vi "RIB Req - UDP Normal Operation.vi"(0 "Limits File Path":path, 5 "Results File Path":path, 11 "error in":errorcluster) -> (4 "Results Data Array":string[][](array[string]), 15 "error out":errorcluster)   [LabVIEW 2024]
doc: "Template test"
uses:
  <vilib>/addons/_JKI Toolkits/State Machine/_JKI_lib_State_Machine.llb/Select State(s)_err__jki_lib_state_machine.vi
  <vilib>/addons/_JKI Toolkits/State Machine/_JKI_lib_State_Machine.llb/Select State(s)_bool__jki_lib_state_machine.vi
  <vilib>/addons/_JKI Toolkits/State Machine/_JKI_lib_State_Machine.llb/Periodic Trigger__ogtk__JKI-SM__jki_lib_state_machine.vi
  <userlib>/_OpenG.lib/file/file.llb/Strip Path Extension - String__ogtk.vi
  <vilib>/Utility/file.llb/Read Delimited Spreadsheet (string).vi
  <userlib>/_OpenG.lib/file/file.llb/openg_file.lvlib
  <userlib>/_OpenG.lib/appcontrol/appcontrol.llb/openg_application_control.lvlib
  <userlib>/_OpenG.lib/time/time.llb/openg_time.lvlib
  <vilib>/Utility/file.llb/Write Delimited Spreadsheet (string).vi
panel:
  in  "Connect":string
  in  "Connect Fail":string
  out "Normal Operation":bool
  out "Wait for Start":bool
  out "Timeout (Normal Operation)":dbl(slide) scale=0.0..10.0
  out "Timeout (Wait for Start)":dbl(slide) scale=0.0..10.0
  in  "Read Normal Operation":string
  in  "Read Wait for Start":string
  in  "Read TMS":string
  in  "Read ROV B":string
  in  "Read ROV A":string
  out "Results Data 10":string[](array[string])
  out "Results Data 9":string[](array[string])
  in  "5A Test":bool
  in  "task out":refnum<k21>
  in  "UDP Read":string
  in  "connection ID":refnum<k16>
  in  "Exit":bool
  # "Normal Operation Test"
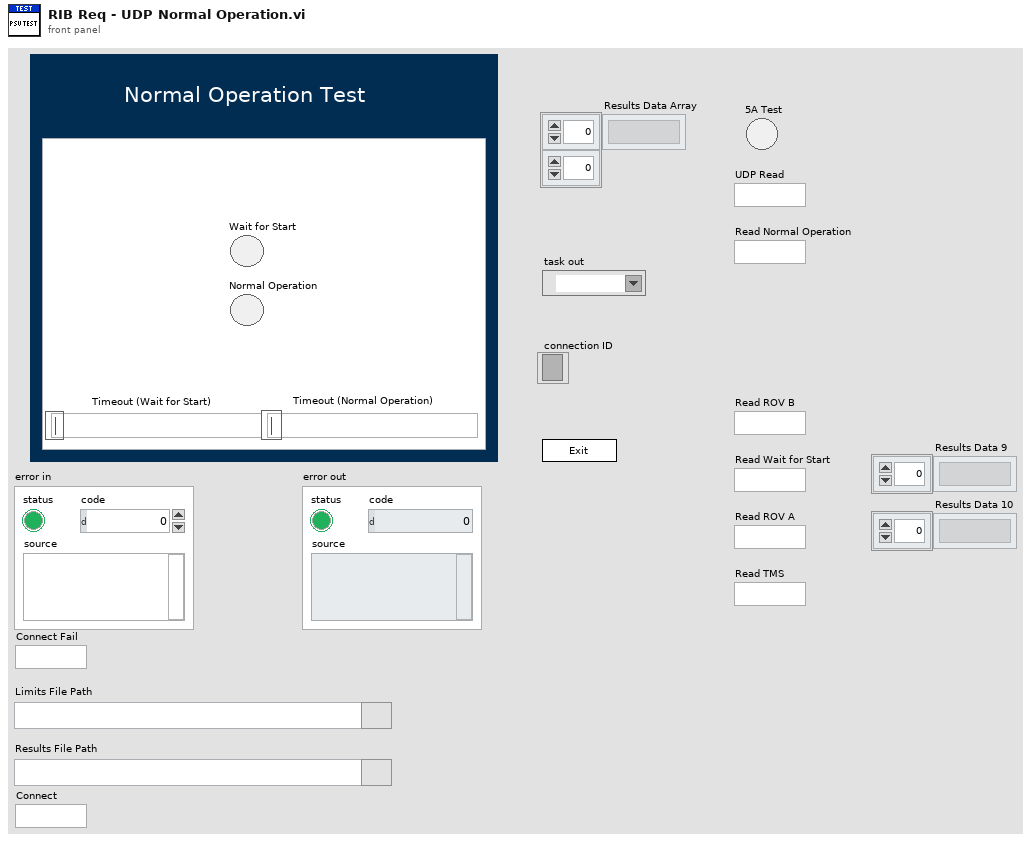
[diagram p1: front panel]
types:
  T1 = enum32{"Invalid", "Standard", "Closed", "Hidden", "Minimized", "Maximized"}
  T2 = enum32{"invalid app kind", "Development System", "Run Time System", "Student Edition", "Embedded LabVIEW", "Evaluation", "Custom"}
  T3 = typedef "FGV - Enum" = enum16{"Cleanup", "Get Data", "Open UDP", "Initialise DAQ", "Initialise I2C"}
  T4 = enum16{"Start Timer", "Get Time", "Pause", "Unpause"}
  T5 = cluster{"Core":cluster{"Current VI Reference":refnum<vi>, "Close Panel on Exit?":bool}, "Limits File Path":path, "Test Limits":string[][], "Results Data Array":string[][], "Results File Path":path, "UDP Read":string, "connection ID":refnum<k16>, "task out":refnum<k21>, "5A Test":bool, "Connect Fail":string, "Connect":string, "Read ROV A":string, "Read ROV B":string, "Read TMS":string, "Read Wait for Start":string, "Read Normal Operation":string}
  T6 = cluster{"Current VI Reference":refnum<vi>, "Close Panel on Exit?":bool}
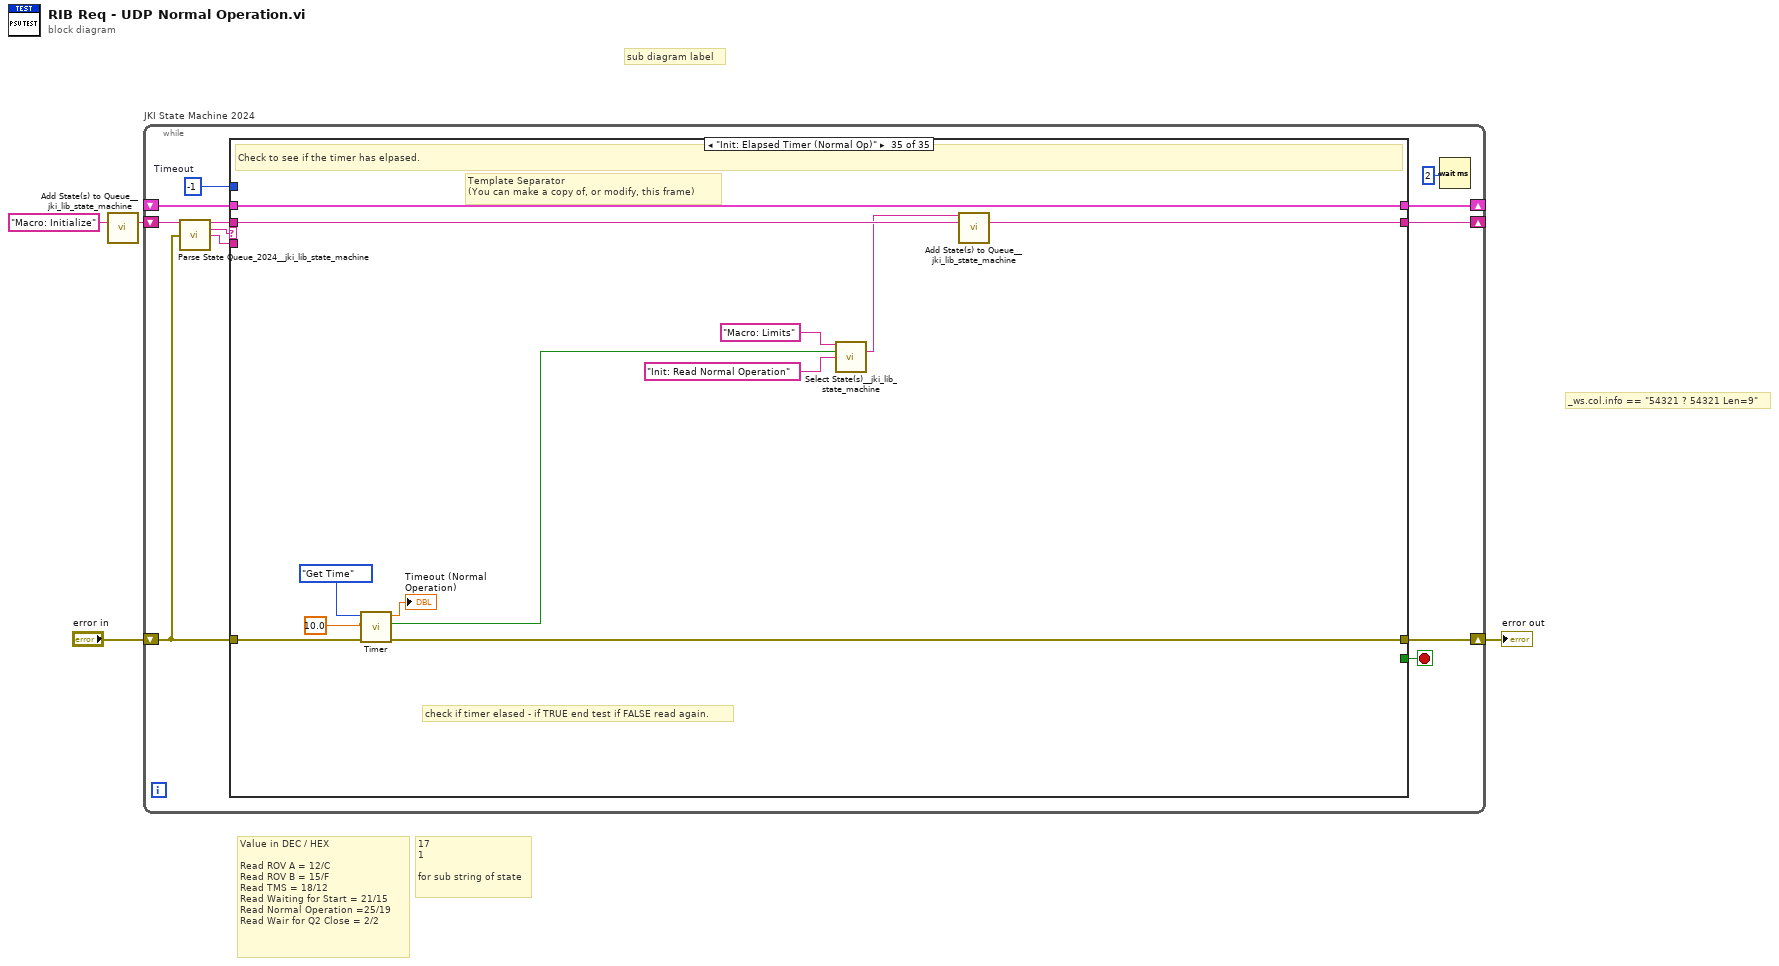
[diagram p0: block diagram]
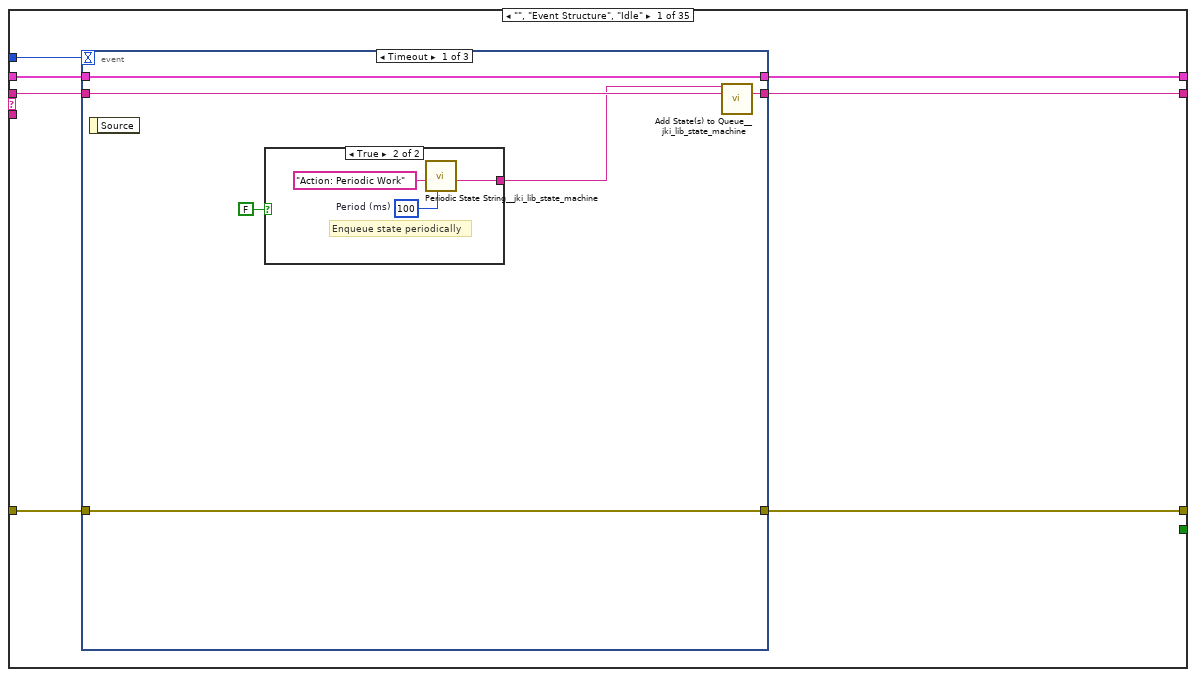
[diagram p2: hidden frame]
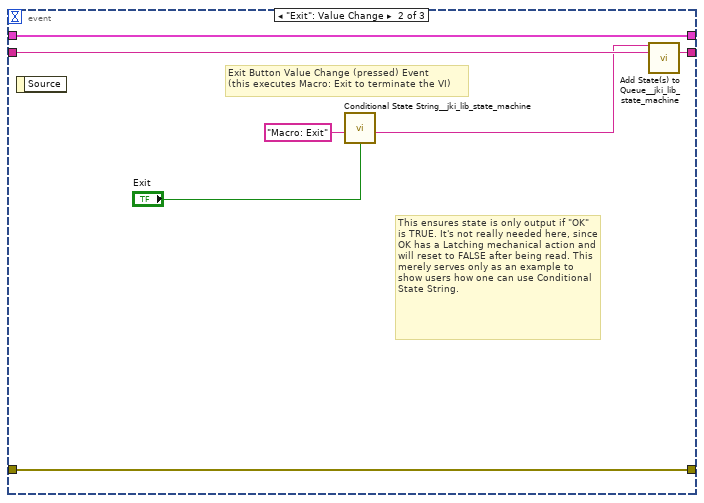
[diagram p4: hidden frame]
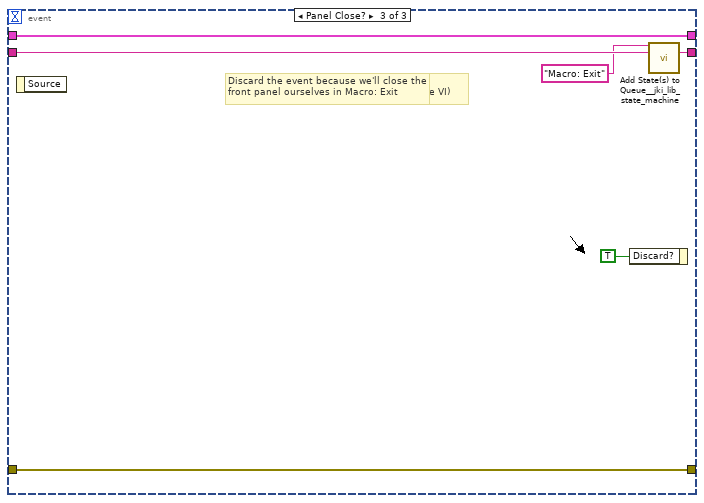
[diagram p5: hidden frame]
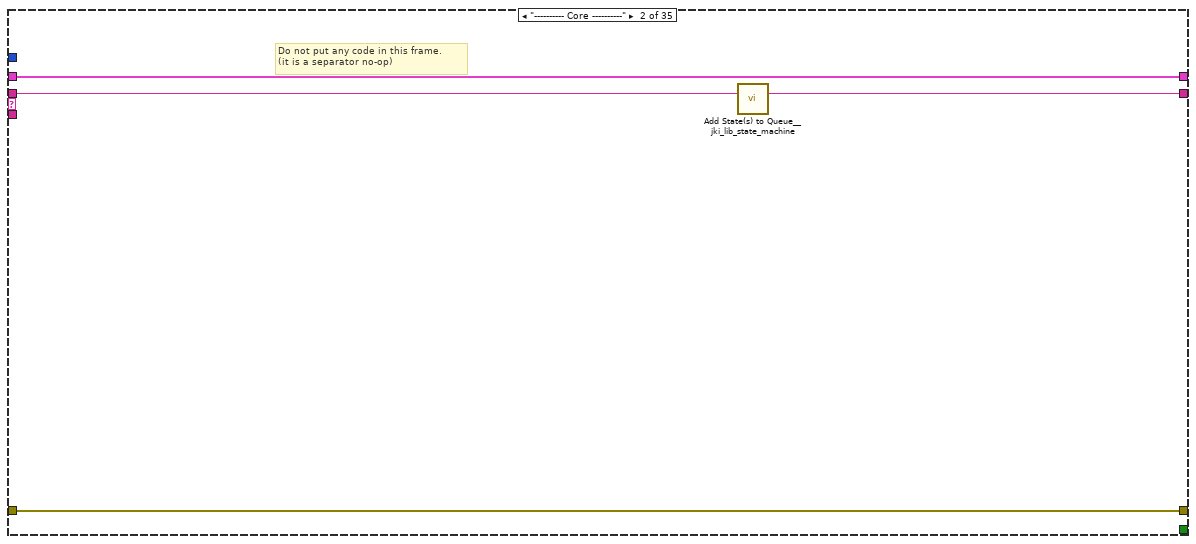
[diagram p6: hidden frame]
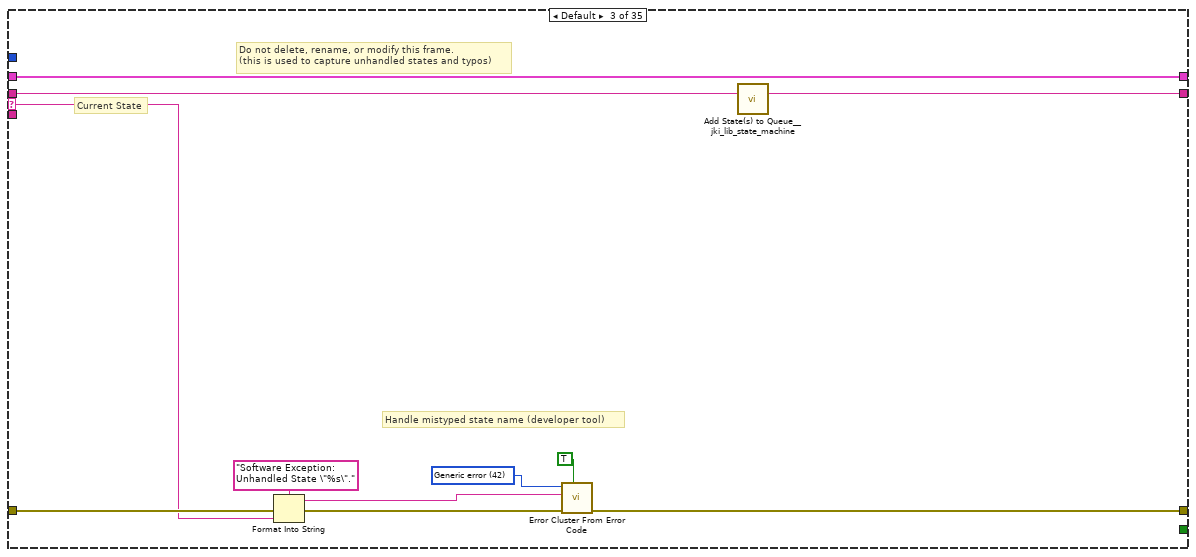
[diagram p7: hidden frame]
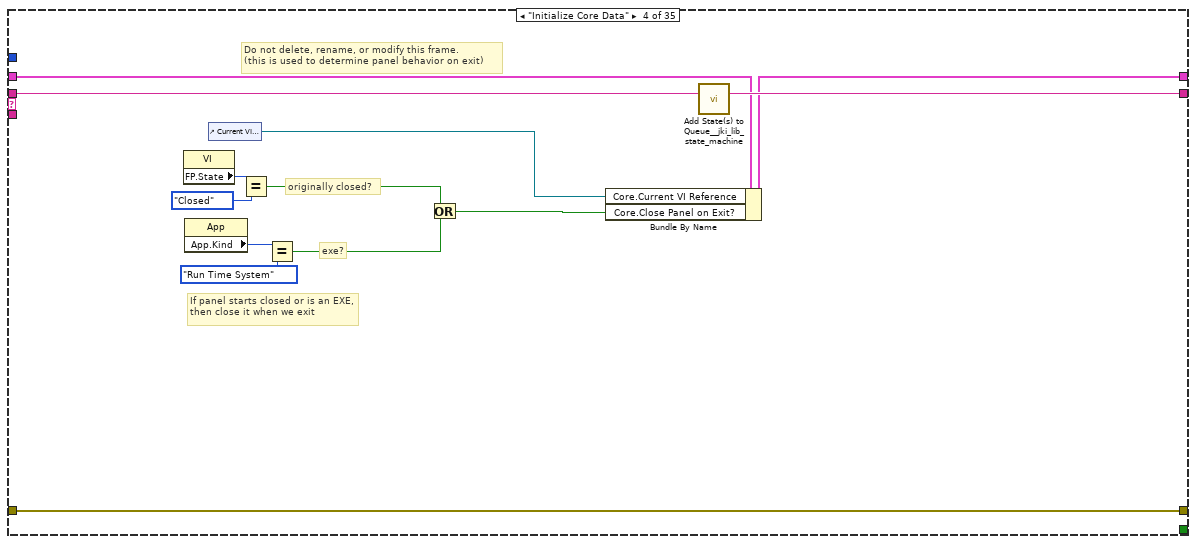
[diagram p8: hidden frame]
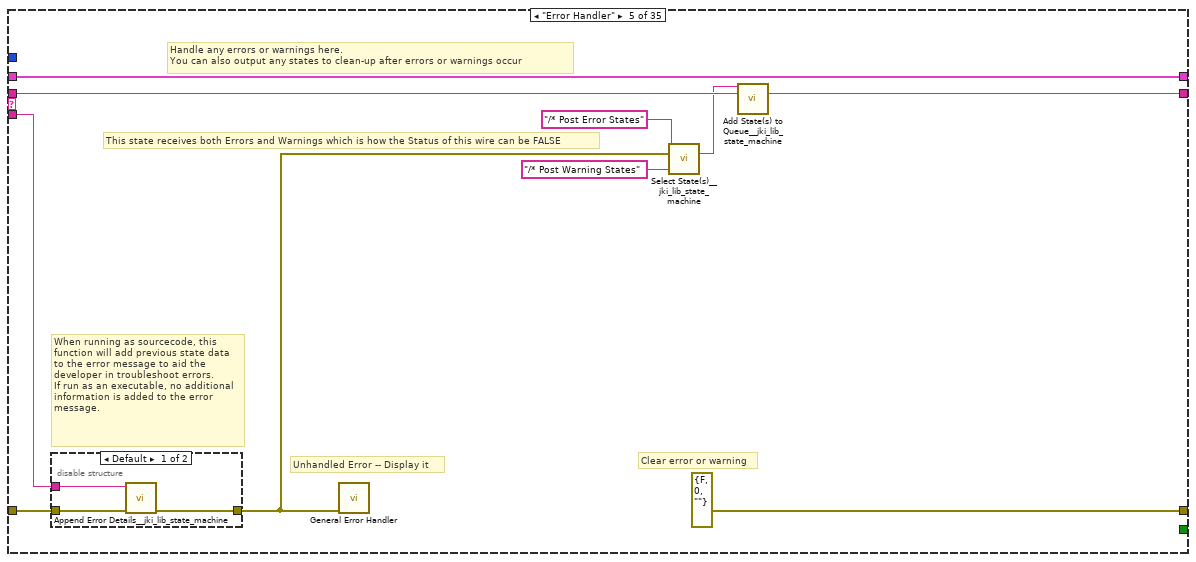
[diagram p9: hidden frame]
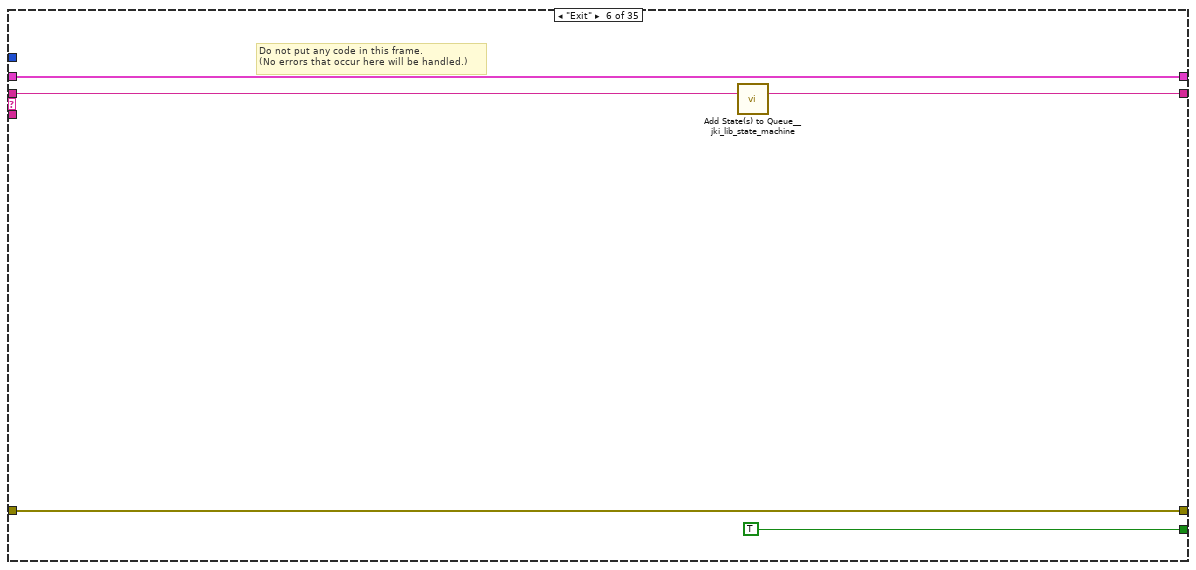
[diagram p11: hidden frame]
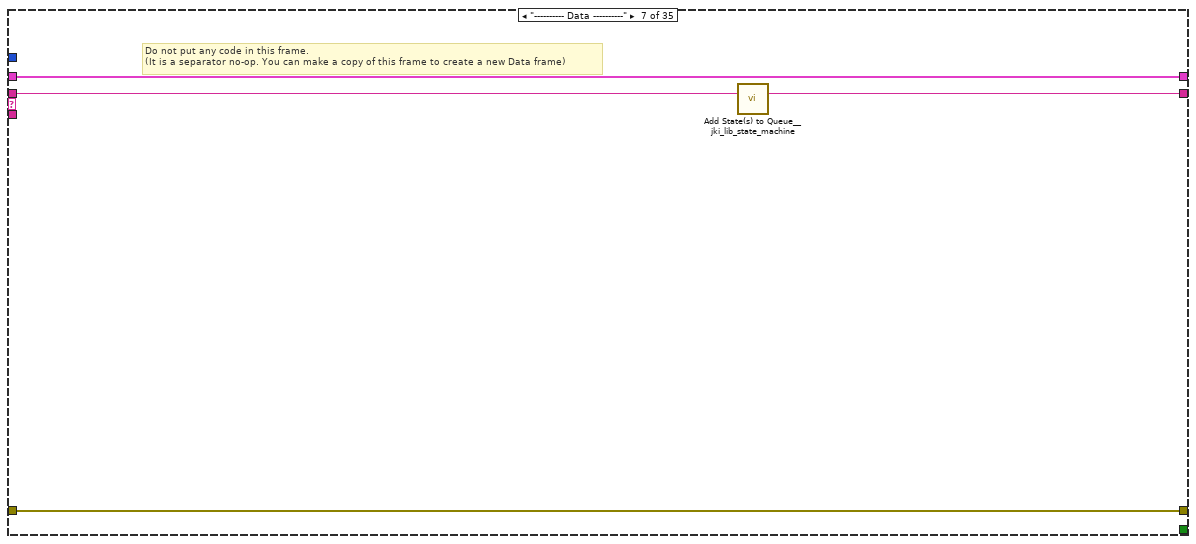
[diagram p12: hidden frame]
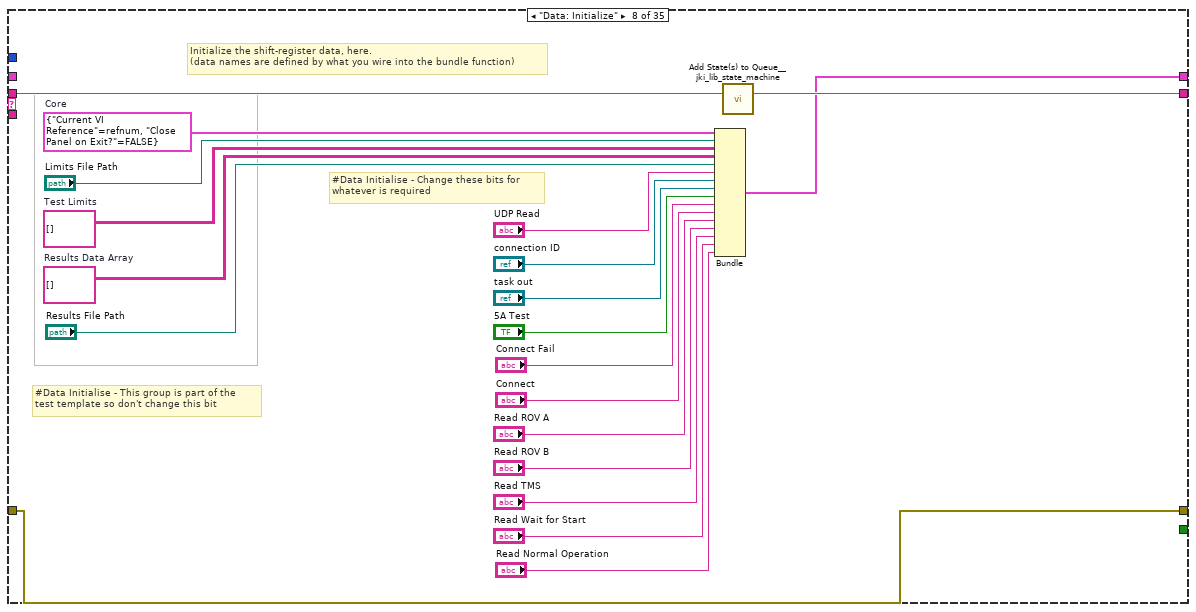
[diagram p13: hidden frame]
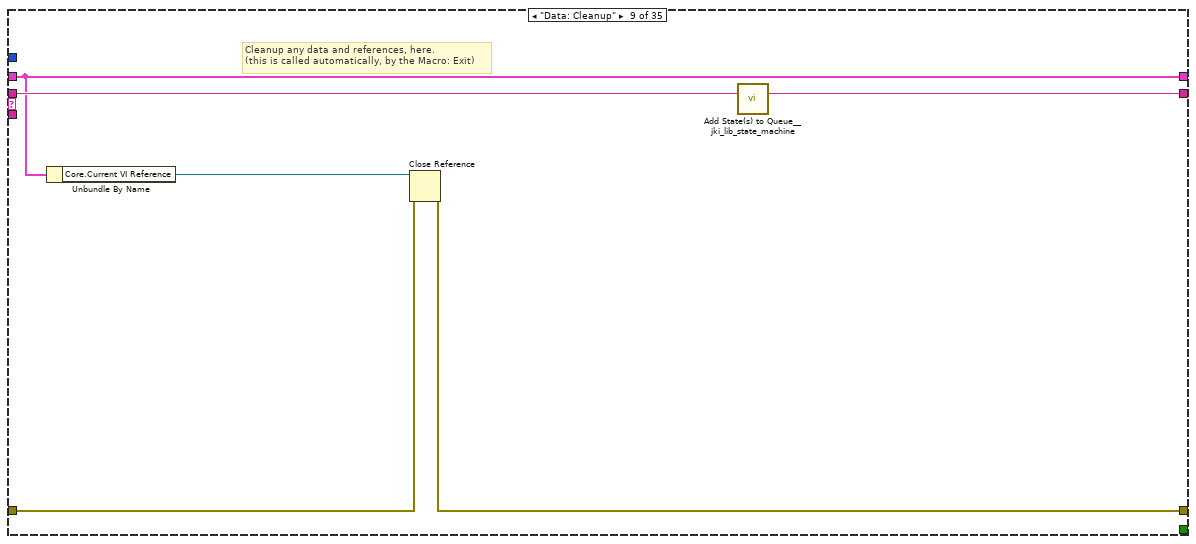
[diagram p14: hidden frame]
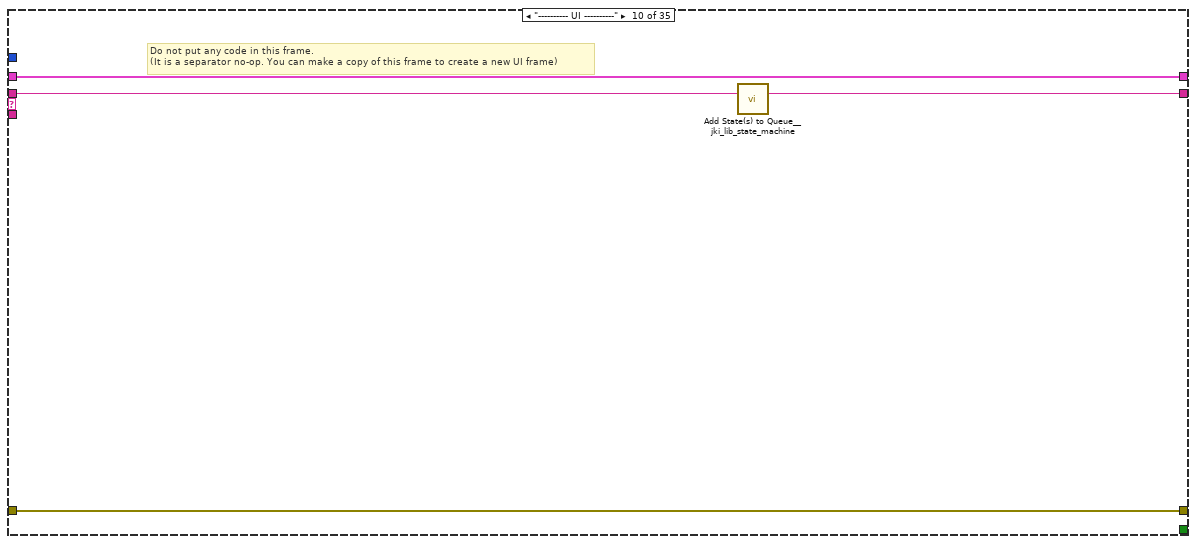
[diagram p15: hidden frame]
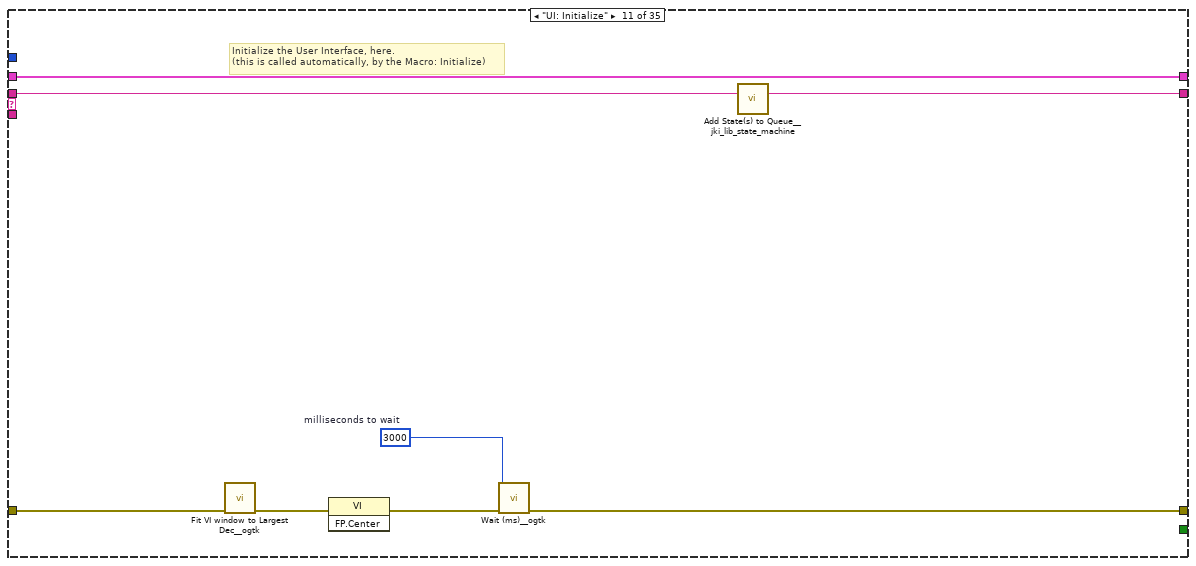
[diagram p16: hidden frame]
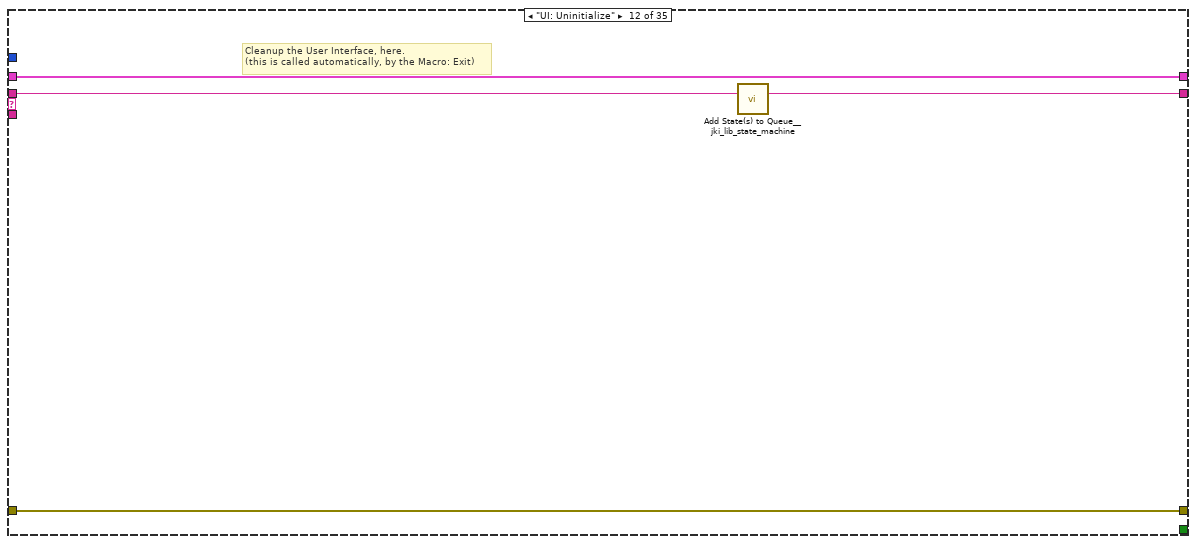
[diagram p17: hidden frame]
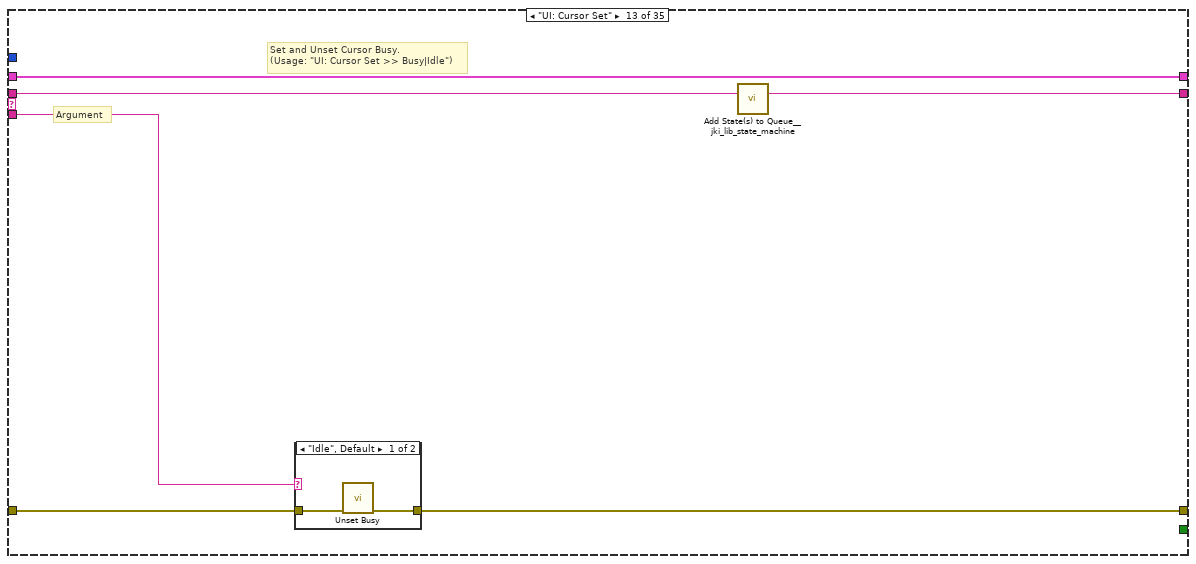
[diagram p18: hidden frame]
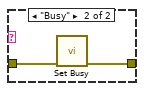
[diagram p19: hidden frame]
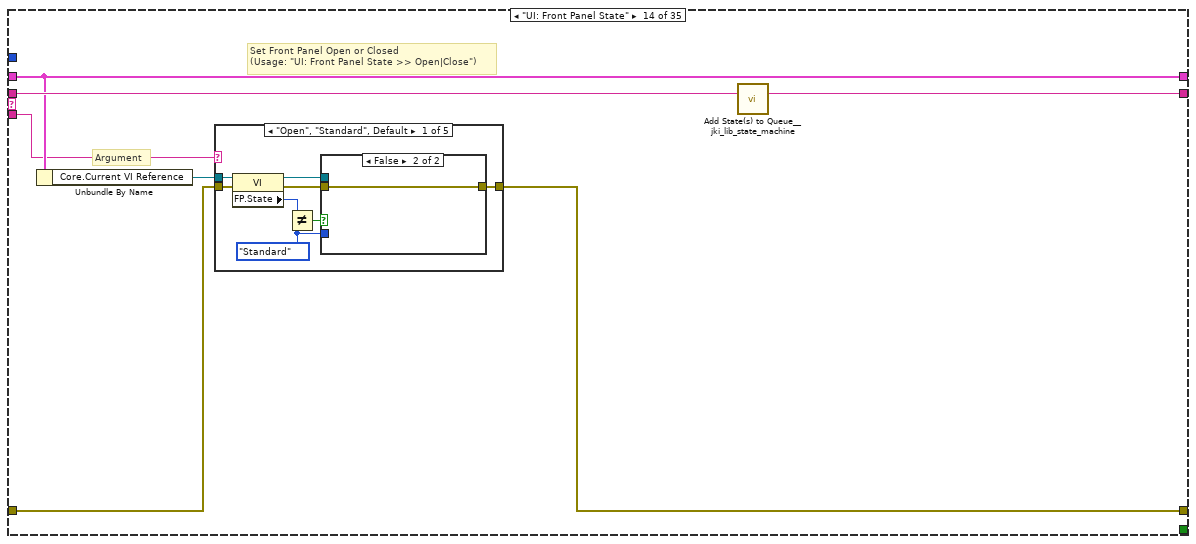
[diagram p20: hidden frame]
diagram:
  # "17\n1\n\nfor sub string of state"
  # "Value in DEC / HEX\n\nRead ROV A = 12/C\nRead ROV B = 15/F\nRead TMS = 18/12\nRead Waiting for Start = 21/15\nRead Normal Operation =25/19 \nRead Wair for Q2 Close = 2/2"
  # "_ws.col.info == \"54321 ? 54321 Len=9\""
  # "sub diagram label"
  n1 = call <vilib>:"Add State(s) to Queue__jki_lib_state_machine.vi"("State(s) in (\"\")"="Macro: Initialize") -> ("States Out"=w4:string)  [unwired: 14 in]
  n2 = while "JKI State Machine 2024" {
    shift-right: [w9] -> _
    shift-left: _ -> [w8]
    shift-right: [w12] -> w1
    shift-left: "error in" -> [w6]
    shift-right: [w11] -> _
    shift-left: w4 -> [w13]
    stop <- w10 stop-if-true
    w7 = -1  # Timeout
    n3 = call <vilib>:"Parse State Queue_2024__jki_lib_state_machine.vi"("State Queue"=w13, "Error In (no error)"=w6) -> ("Remaining States"=w15:string, "Current State"=w16:string, "Arguments"=w14:string)  [unwired: 11 in]
    n4 = case shown="\"Init: Elapsed Timer (Normal Op)\"" w16 {
      selector: w16 -> [_ _ w50 _ _ _ _ _ _ _ _ _ _ _ _ _ _ _ _ _ _ _ _ _ _ _ _ _ _ _ _ _ _ _ _]
      tunnel: w15 -> [w23 w49 w54 w73 w83 w92 w96 w116 w122 w126 w134 w138 w144 w155 w224 w229 w234 w239 w244 w253 w257 w270 w287 w300 w304 w313 w317 w325 w336 w360 w372 w393 w404 w428 w440]
      tunnel: w14 -> [_ _ _ _ w78 _ _ _ _ _ _ _ w139 w149 _ _ _ _ _ _ _ _ _ _ _ _ _ _ _ _ _ _ _ _ _]
      tunnel: w8 -> [w21 w46 w52 w66 w80 w90 w93 _ w117 w123 w132 w136 w142 w151 w221 w226 w231 w236 w241 w251 w254 w260 w279 w292 w301 w309 w314 w323 w334 w343 w370 w390 w402 w423 w438]
      tunnel: [w20 w47 w56 w70 errorcluster {"status"=FALSE, "code"=0, "source"=""} ("error out") w89 w94 w113 w118 w124 w130 w135 w140 w152 w222 w227 w232 w237 w242 w248 w255 w266 w284 w297 w302 w311 w315 w320 w329 w339 w367 w374 w398 w421 w435] -> w12
      tunnel: w6 -> [w17 w47 w55 w70 w79 w89 w94 w113 w119 w124 w131 w135 w141 w153 w222 w227 w232 w237 w242 w248 w255 w265 w283 w296 w302 w310 w315 w318 w332 w338 w368 w379 w400 w422 w436]
      tunnel: [w22 w48 w53 w72 w82 w91 w95 w115 w121 w125 w133 w137 w143 w154 w223 w228 w233 w238 w243 w252 w256 w269 w286 w299 w303 w312 w316 w324 w335 w359 w371 w392 w403 w427 w439] -> w11
      tunnel: [_ _ _ _ _ TRUE _ _ _ _ _ _ _ _ _ _ _ _ _ _ _ _ _ _ _ _ _ _ _ _ _ _ _ _ _] -> w10
      tunnel: [w19 w46 w52 w71 w80 w90 w93 w114 w117 w123 w132 w136 w142 w151 w221 w226 w231 w236 w241 w251 w254 w259 w278 w291 w301 w309 w314 w322 w334 w342 w370 w391 w402 w420 w438] -> w9
      tunnel: w7 -> [w18 _ _ _ _ _ _ _ _ _ _ _ _ _ _ _ _ _ _ _ _ _ _ _ _ _ _ _ _ _ _ _ _ _ _]
      frame "", "Event Structure", "Idle" {
        n5 = event shown="[0] Timeout" {
          selector: _ -> [_ _ _]
          dyn-events: _ -> [_ _ _]
          timeout: w18 -> [_ _ _]
          tunnel: w23 -> [w29 w39 w45]
          tunnel: [w28 w38 w44] -> w22
          tunnel: w21 -> [w26 w36 w42]
          tunnel: [w27 w37 w43] -> w20
          tunnel: w17 -> [w27 w37 w43]
          tunnel: [w26 w36 w42] -> w19
          event Timeout {
            n6 = event-data() -> ()  [unwired: 1 in, 1 out]
            n7 = case shown="True" FALSE {
              tunnel: [_ w32] -> w25
              frame False {
              }
              frame True {
                w30 = u32 100  # Period (ms)
                # "Enqueue state periodically"
                n8 = call <vilib>:"Periodic State String__jki_lib_state_machine.vi"("Period (ms)"=w30, "State"="Action: Periodic Work") -> ("State Out"=w32:string)  [unwired: 9 in]
              }
            }
            n9 = call <vilib>:"Add State(s) to Queue__jki_lib_state_machine.vi"("State(s) in Front (\"\")"=w25, "State(s) in (\"\")"=w29) -> ("States Out"=w28:string)  [unwired: 13 in]
          }
          event "Exit": Value Change {
            # "This ensures state is only output if \"OK\" is TRUE. It's not really needed here, since OK has a Latching mechanical action and will reset to FALSE after being read. This merely serves only as an example to show users how one can use Conditional State String."
            # "Exit Button Value Change (pressed) Event\n(this executes Macro: Exit to terminate the VI)"
            n10 = event-data() -> ()  [unwired: 1 in, 1 out]
            n11 = call <vilib>:"Conditional State String__jki_lib_state_machine.vi"("Do State(s)?"="Exit", "State"="Macro: Exit") -> ("State Out"=w33:string)  [unwired: 7 in]
            n12 = call <vilib>:"Add State(s) to Queue__jki_lib_state_machine.vi"("State(s) in Front (\"\")"=w33, "State(s) in (\"\")"=w39) -> ("States Out"=w38:string)  [unwired: 13 in]
          }
          event Panel Close? {
            # "Discard the event because we'll close the front panel ourselves in Macro: Exit"
            # "Close Panel button (pressed) Event\n(this executes Macro: Exit to terminate the VI)"
            n13 = event-data() -> ()  [unwired: 1 in, 1 out]
            n14 = event-data("Discard?"=TRUE) -> ()  [unwired: 1 in, 1 out]
            n15 = call <vilib>:"Add State(s) to Queue__jki_lib_state_machine.vi"("State(s) in Front (\"\")"="Macro: Exit", "State(s) in (\"\")"=w45) -> ("States Out"=w44:string)  [unwired: 13 in]
          }
        }
      }
      frame "---------- Core ----------" {
        # "Do not put any code in this frame.\n(it is a separator no-op)"
        n16 = call <vilib>:"Add State(s) to Queue__jki_lib_state_machine.vi"("State(s) in (\"\")"=w49) -> ("States Out"=w48:string)  [unwired: 14 in]
      }
      frame Default {
        w59 = 42 items=["No error", "Argument error", "Memory is full", "Out of zone", "End of file", "File already open", "Generic file I/O error", "File not found", "File permission error", "Disk is full", "Duplicate path", "Too many files open", "System feature not enabled", "Resource file not found", "Cannot add resource", "Resource not found", "Image not found", "Image memory error", "Pen does not exist", "Config type invalid", "Config token not found", "Config parse error", "Config memory error", "Bad external code format", "Bad external code offset", "External code not present", "Null window", "Destroy window error", "Null menu", "Print aborted", "Bad print record", "Print driver error", "Windows error during printing", "Memory error during printing", "Print dialog error", "Generic print error", "Invalid device refnum", "Device not found", "Device parameter error", "Device unit error", "Cannot open device", "Device call aborted", "Generic error", "Cancelled by user", "Object ID too low", "Object ID too high", "Object not in heap", "Unknown heap", "Unknown object (invalid DefProc)", "Unknown object (DefProc not in table)", "Message out of range", "Invalid (null) method", "Unknown message", "Manager call not supported", "Bad address", "Network operation in progress", "Network operation timed out", "Connection is busy", "Network attribute not supported", "Network error", "Address in use", "System out of memory", "Connection aborted", "Connection refused", "Not connected", "Already connected", "Connection closed", "Initialization error (interapplication manager)", "Bad occurrence", "Wait on unbound occurrence handler", "Occurrence queue overflow", "Datalog type conflict", "Unused", "Unrecognized type (interapplication manager)", "Memory corrupt", "Failed to make temporary DLL", "Old CIN version", "Drag socket not found", "Failed to load drop-object", "Failed to register OLE object", "Failed to release OLE object", "Format specifier type mismatch", "Unknown format specifier", "Too few format specifiers", "Too many format specifiers", "Scan failed", "Newer CIN version", "Error converting to variant", "Runtime menu error", "Password tampered", "Variant attribute not found", "Incompatible variant data type", "Event data is not available", "Event Store is not present", "Occurrence is not found", "Event Queue is not created", "Event info is not available", "Refnum passed is NULL", "Error retrieving Class GUID", "Error retrieving CoClass GUID", "Error retrieving TypeLib GUID.", "Bad built application magic bytes.", "Specific driver is different from the specific driver associated with the Logical Name.", "There is no session opened to the class driver.", "Max Error", "MAX - Error with config objects", "MAX - Error loading configuration", "MAX - Group not supported"]
        # "Current State"
        # "Do not delete, rename, or modify this frame.\n(this is used to capture unhandled states and typos)"
        # "Handle mistyped state name (developer tool)"
        n17 = Format Into String(format string="Software Exception: Unhandled State \"%s\"." ("message"), error in=w55, w50) -> (resulting string=w58:string, error out=w57:errorcluster)  [unwired: 1 in]
        n18 = call <vilib>:"Error Cluster From Error Code.vi"("show call chain? (False)"=TRUE, "error in (no error)"=w57, "error message (\"\")"=w58, "error code (0)"=w59) -> ("error out"=w56:errorcluster)  [unwired: 5 in]
        n19 = call <vilib>:"Add State(s) to Queue__jki_lib_state_machine.vi"("State(s) in (\"\")"=w54) -> ("States Out"=w53:string)  [unwired: 14 in]
      }
      frame "Initialize Core Data" {
        # "Do not delete, rename, or modify this frame.\n(this is used to determine panel behavior on exit)"
        # "originally closed?"
        # "exe?"
        # "If panel starts closed or is an EXE, then close it when we exit"
        n20 = property class="VI"() -> ("FP.State"=w63:T1)  [unwired: 2 in, 2 out]
        n21 = property class="App"() -> ("App.Kind"=w69:T2)  [unwired: 2 in, 2 out]
        n22 = control-ref of="Current VI Reference"() -> (w64:refnum<vi>)
        n23 = Equal?(x=w63, y=T1."Closed" ("Front Panel Window:State")) -> (x = y?=w61:bool)
        n24 = Equal?(x=w69, y=T2."Run Time System" ("Application:Kind")) -> (x = y?=w67:bool)
        n25 = Or(x=w61, y=w67) -> (x .or. y?=w65:bool)
        n26 = Bundle By Name(cluster=w66, "Core.Current VI Reference"=w64, "Core.Close Panel on Exit?"=w65) -> (w71:T5)
        n27 = call <vilib>:"Add State(s) to Queue__jki_lib_state_machine.vi"("State(s) in (\"\")"=w73) -> ("States Out"=w72:string)  [unwired: 14 in]
      }
      frame "Error Handler" {
        # "When running as sourcecode, this function will add previous state data to the error message to aid the developer in troubleshoot errors.\nIf run as an executable, no additional information is added to the error message."
        # "This state receives both Errors and Warnings which is how the Status of this wire can be FALSE"
        # "Unhandled Error -- Display it"
        # "Handle any errors or warnings here.\nYou can also output any states to clean-up after errors or warnings occur"
        # "Clear error or warning"
        n28 = disable-structure shown="Default" {
          disable-tunnel: w79 -> [w86 w87]
          disable-tunnel: w78 -> [w85 _]
          disable-tunnel: [w84 w87] -> w77
          frame condition #0 (active) {
            n29 = call <vilib>:"Append Error Details__jki_lib_state_machine.vi"("error in (no error)"=w86, "Previous State and Argument(s)"=w85) -> ("error out"=w84:errorcluster)  [unwired: 9 in]
          }
          frame condition #1 {
          }
        }
        n30 = call <vilib>:"General Error Handler.vi"("error in (no error)"=w77) -> ()  [unwired: 10 in, 5 out]
        n31 = call-poly <vilib>:"Select State(s)__jki_lib_state_machine.vi"("State(s) if True (\"\")"="/* Post Error States", "Select"=w77, "State(s) if False (\"\")"="/* Post Warning States") -> ("States Out"=w75:string)  [unwired: 12 in]
        n32 = call <vilib>:"Add State(s) to Queue__jki_lib_state_machine.vi"("State(s) in Front (\"\")"=w75, "State(s) in (\"\")"=w83) -> ("States Out"=w82:string)  [unwired: 13 in]
      }
      frame "Exit" {
        # "Do not put any code in this frame.\n(No errors that occur here will be handled.)"
        n33 = call <vilib>:"Add State(s) to Queue__jki_lib_state_machine.vi"("State(s) in (\"\")"=w92) -> ("States Out"=w91:string)  [unwired: 14 in]
      }
      frame "---------- Data ----------" {
        # "Do not put any code in this frame.\n(It is a separator no-op. You can make a copy of this frame to create a new Data frame)"
        n34 = call <vilib>:"Add State(s) to Queue__jki_lib_state_machine.vi"("State(s) in (\"\")"=w96) -> ("States Out"=w95:string)  [unwired: 14 in]
      }
      frame "Data: Initialize" {
        w109 = string[][] []  # Results Data Array
        w110 = string[][] []  # Test Limits
        w112 = T6 {"Current VI Reference"=refnum, "Close Panel on Exit?"=FALSE}  # Core
        # "#Data Initialise - Change these bits for\nwhatever is required"
        # "#Data Initialise - This group is part of the\ntest template so don't change this bit"
        # "Initialize the shift-register data, here.\n(data names are defined by what you wire into the bundle function)"
        n35 = Bundle("Core"=w112, "Limits File Path"="Limits File Path", "Test Limits"=w110, "Results Data Array"=w109, "Results File Path"="Results File Path", "UDP Read"="UDP Read", "connection ID"="connection ID", "task out"="task out", "5A Test"="5A Test", "Connect Fail"="Connect Fail", "Connect"="Connect", "Read ROV A"="Read ROV A", "Read ROV B"="Read ROV B", "Read TMS"="Read TMS", "Read Wait for Start"="Read Wait for Start", "Read Normal Operation"="Read Normal Operation") -> (w114:T5)  [unwired: 1 in]
        n36 = call <vilib>:"Add State(s) to Queue__jki_lib_state_machine.vi"("State(s) in (\"\")"=w116) -> ("States Out"=w115:string)  [unwired: 14 in]
      }
      frame "Data: Cleanup" {
        # "Cleanup any data and references, here.\n(this is called automatically, by the Macro: Exit)"
        n37 = Unbundle By Name(w117) -> ("Core.Current VI Reference"=w120:refnum<vi>)
        n38 = Close Reference(reference=w120, error in (no error)=w119) -> (error out=w118:errorcluster)
        n39 = call <vilib>:"Add State(s) to Queue__jki_lib_state_machine.vi"("State(s) in (\"\")"=w122) -> ("States Out"=w121:string)  [unwired: 14 in]
      }
      frame "---------- UI ----------" {
        # "Do not put any code in this frame.\n(It is a separator no-op. You can make a copy of this frame to create a new UI frame)"
        n40 = call <vilib>:"Add State(s) to Queue__jki_lib_state_machine.vi"("State(s) in (\"\")"=w126) -> ("States Out"=w125:string)  [unwired: 14 in]
      }
      frame "UI: Initialize" {
        w129 = u32 3000  # milliseconds to wait
        # "Initialize the User Interface, here.\n(this is called automatically, by the Macro: Initialize)"
        n41 = call <userlib>:"Fit VI window to Largest Dec__ogtk.vi"("error in (no error)"=w131) -> ("error out"=w127:errorcluster)  [unwired: 5 in, 1 out]
        n42 = invoke class="VI" method="FP.Center"(error in=w127) -> (error out=w128:errorcluster)  [unwired: 2 in, 2 out]
        n43 = call <userlib>:"Wait (ms)__ogtk.vi"("error in (no error)"=w128, "milliseconds to wait"=w129) -> ("error out"=w130:errorcluster)  [unwired: 8 in, 1 out]
        n44 = call <vilib>:"Add State(s) to Queue__jki_lib_state_machine.vi"("State(s) in (\"\")"=w134) -> ("States Out"=w133:string)  [unwired: 14 in]
      }
      frame "UI: Uninitialize" {
        # "Cleanup the User Interface, here.\n(this is called automatically, by the Macro: Exit)"
        n45 = call <vilib>:"Add State(s) to Queue__jki_lib_state_machine.vi"("State(s) in (\"\")"=w138) -> ("States Out"=w137:string)  [unwired: 14 in]
      }
      frame "UI: Cursor Set" {
        # "Argument"
        # "Set and Unset Cursor Busy.\n(Usage: \"UI: Cursor Set >> Busy|Idle\")"
        n46 = case shown="\"Idle\", Default" w139 {
          tunnel: w141 -> [w146 w148]
          tunnel: [w145 w147] -> w140
          frame "Idle", Default {
            n47 = call <vilib>:"Unset Busy.vi"("error in (no error)"=w146) -> ("error out"=w145:errorcluster)  [unwired: 10 in]
          }
          frame "Busy" {
            n48 = call <vilib>:"Set Busy.vi"("error in (no error)"=w148) -> ("error out"=w147:errorcluster)  [unwired: 9 in, 1 out]
          }
        }
        n49 = call <vilib>:"Add State(s) to Queue__jki_lib_state_machine.vi"("State(s) in (\"\")"=w144) -> ("States Out"=w143:string)  [unwired: 14 in]
      }
      frame "UI: Front Panel State" {
        # "Argument"
        # "Set Front Panel Open or Closed\n(Usage: \"UI: Front Panel State >> Open|Close\")"
        n50 = Unbundle By Name(w151) -> ("Core.Current VI Reference"=w150:refnum<vi>)
        n51 = case shown="\"Open\", \"Standard\", Default" w149 {
          tunnel: w153 -> [w161 w176 w187 w200 w213]
          tunnel: [w163 w177 w189 w202 w215] -> w152
          tunnel: w150 -> [w162 w174 w188 w201 w214]
          frame "Open", "Standard", Default {
            w156 = T1."Standard" ("State")
            n52 = property class="VI"(reference=w162, error in=w161) -> (reference out=w159:refnum<vi>, error out=w160:errorcluster, "FP.State"=w158:T1)
            n53 = Not Equal?(x=w158, y=w156) -> (x != y?=w157:bool)
            n54 = case shown="False" w157 {
              tunnel: [w167 w169] -> w163
              tunnel: w160 -> [w166 w169]
              tunnel: w159 -> [w165 _]
              tunnel: w156 -> [w164 _]
              frame True {
                n55 = invoke class="VI" method="FP.Open"(reference=w165, error in=w166, "Activate"=TRUE, "State"=w164) -> (error out=w167:errorcluster)  [unwired: 1 in, 4 out]
              }
              frame False {
              }
            }
          }
          frame "Close", "Closed" {
            n56 = property class="VI"(reference=w174, error in=w176) -> (reference out=w173:refnum<vi>, error out=w175:errorcluster, "FP.State"=w171:T1)
            n57 = Not Equal?(x=w171, y=T1."Closed" ("Front Panel Window:State")) -> (x != y?=w170:bool)
            n58 = case shown="True" w170 {
              tunnel: [w178 w181] -> w177
              tunnel: w175 -> [w178 w180]
              tunnel: w173 -> [_ w179]
              frame False {
              }
              frame True {
                n59 = invoke class="VI" method="FP.Close"(reference=w179, error in=w180) -> (error out=w181:errorcluster)  [unwired: 1 in, 2 out]
              }
            }
          }
          frame "Hidden", "Hide" {
            w182 = T1."Hidden" ("State")
            n60 = property class="VI"(reference=w188, error in=w187) -> (reference out=w185:refnum<vi>, error out=w186:errorcluster, "FP.State"=w184:T1)
            n61 = Not Equal?(x=w184, y=w182) -> (x != y?=w183:bool)
            n62 = case shown="True" w183 {
              tunnel: [w193 w194] -> w189
              tunnel: w186 -> [w192 w194]
              tunnel: w185 -> [w191 _]
              tunnel: w182 -> [w190 _]
              frame True {
                n63 = invoke class="VI" method="FP.Open"(reference=w191, error in=w192, "State"=w190) -> (error out=w193:errorcluster)  [unwired: 2 in, 4 out]
              }
              frame False {
              }
            }
          }
          frame "Minimize", "Minimized" {
            w195 = T1."Minimized" ("State")
            n64 = property class="VI"(reference=w201, error in=w200) -> (reference out=w198:refnum<vi>, error out=w199:errorcluster, "FP.State"=w197:T1)
            n65 = Not Equal?(x=w197, y=w195) -> (x != y?=w196:bool)
            n66 = case shown="True" w196 {
              tunnel: [w206 w207] -> w202
              tunnel: w199 -> [w205 w207]
              tunnel: w198 -> [w204 _]
              tunnel: w195 -> [w203 _]
              frame True {
                n67 = invoke class="VI" method="FP.Open"(reference=w204, error in=w205, "State"=w203) -> (error out=w206:errorcluster)  [unwired: 2 in, 4 out]
              }
              frame False {
              }
            }
          }
          frame "Maximize", "Maximized" {
            w208 = T1."Maximized" ("State")
            n68 = property class="VI"(reference=w214, error in=w213) -> (reference out=w211:refnum<vi>, error out=w212:errorcluster, "FP.State"=w210:T1)
            n69 = Not Equal?(x=w210, y=w208) -> (x != y?=w209:bool)
            n70 = case shown="True" w209 {
              tunnel: [w219 w220] -> w215
              tunnel: w212 -> [w218 w220]
              tunnel: w211 -> [w217 _]
              tunnel: w208 -> [w216 _]
              frame True {
                n71 = invoke class="VI" method="FP.Open"(reference=w217, error in=w218, "State"=w216) -> (error out=w219:errorcluster)  [unwired: 2 in, 4 out]
              }
              frame False {
              }
            }
          }
        }
        n72 = call <vilib>:"Add State(s) to Queue__jki_lib_state_machine.vi"("State(s) in (\"\")"=w155) -> ("States Out"=w154:string)  [unwired: 14 in]
      }
      frame "---------- Macro ----------" {
        # "Do not put any code in this frame.\n(It is a separator no-op. You can make a copy of this frame to create a new Macro frame)"
        n73 = call <vilib>:"Add State(s) to Queue__jki_lib_state_machine.vi"("State(s) in (\"\")"=w224) -> ("States Out"=w223:string)  [unwired: 14 in]
      }
      frame "Macro: Initialize" {
        # "Initialization Macro\n(This is called once, when the VI starts)"
        n74 = call <vilib>:"Add State(s) to Queue__jki_lib_state_machine.vi"("State(s) in Front (\"\")"="Data: Initialize\nInitialize Core Data\nUI: Initialize\nUI: Front Panel State >> Open\nMacro: Test", "State(s) in (\"\")"=w229) -> ("States Out"=w228:string)  [unwired: 13 in]
      }
      frame "Macro: Test" {
        # "#Test Macro - Add the sequence \nfor measurments and limits testing here"
        n75 = call <vilib>:"Add State(s) to Queue__jki_lib_state_machine.vi"("State(s) in Front (\"\")"="Limits Test: Read Limits File\nInit: UDP Open\nInit: Start Timer (WfS)\nInit: Read Wait for Start State", "State(s) in (\"\")"=w234) -> ("States Out"=w233:string)  [unwired: 13 in]
      }
      frame "Macro: Test 2" {
        # "#Test Macro - Add the sequence \nfor measurments and limits testing here"
        n76 = call <vilib>:"Add State(s) to Queue__jki_lib_state_machine.vi"("State(s) in Front (\"\")"="Init: Start Command\nInit: Start Timer (Normal Op)\nInit: Read Normal Operation", "State(s) in (\"\")"=w239) -> ("States Out"=w238:string)  [unwired: 13 in]
      }
      frame "Macro: Limits" {
        # "Do not put any code in this frame.\n(It is a separator no-op. You can make a copy of this frame to create a new Macro frame)"
        n77 = call <vilib>:"Add State(s) to Queue__jki_lib_state_machine.vi"("State(s) in Front (\"\")"="Limits Test: Read Wait for Start Test\nLimits Test: Read Normal Operation Test\nResults Data: Write Results Data\nMacro: Exit", "State(s) in (\"\")"=w244) -> ("States Out"=w243:string)  [unwired: 13 in]
      }
      frame "Macro: Exit" {
        # "Exit Macro\n(This is called once, when the VI exits)"
        n78 = Unbundle By Name(w251) -> ("Core.Close Panel on Exit?"=w246:bool)
        n79 = call <vilib>:"Conditional State String__jki_lib_state_machine.vi"("Do State(s)?"=w246, "State"="UI: Front Panel State >> Close") -> ("State Out"=w245:string)  [unwired: 7 in]
        n80 = call <vilib>:"Add State(s) to Queue__jki_lib_state_machine.vi"("State(s) in (\"\")"=w245, "State(s) at Back (\"\")"="UI: Uninitialize\nData: Cleanup\nExit") -> ("States Out"=w249:string)  [unwired: 13 in]
        n81 = call <vilib>:"Add State(s) to Queue__jki_lib_state_machine.vi"("State(s) in Front (\"\")"=w249, "State(s) in (\"\")"=w253) -> ("States Out"=w252:string)  [unwired: 13 in]
      }
      frame "---------- Limits Test ----------" {
        # "Template Separator\n(You can make a copy of, or modify, this frame)"
        n82 = call <vilib>:"Add State(s) to Queue__jki_lib_state_machine.vi"("State(s) in (\"\")"=w257) -> ("States Out"=w256:string)  [unwired: 14 in]
      }
      frame "Limits Test: Read Limits File" {
        w263 = ","  # delimiter (\t)
        n83 = Unbundle By Name(w260) -> ("Limits File Path"=w264:path)
        n84 = Current VI's Path "Test Case Path"() -> (path=w268:path)
        n85 = call-poly <vilib>:"Read Delimited Spreadsheet.vi"("file path (dialog if empty)"=w264, "error in (no error)"=w265, "delimiter (\\t)"=w263) -> ("all rows"=w261:string[][], "error out"=w266:errorcluster)  [unwired: 7 in, 4 out]
        n86 = Strip Path(path=w268) -> (name=w267:string)  [unwired: 1 out]
        n87 = call-poly <userlib>:"Strip Path Extension__ogtk.vi"("path"=w267) -> ("root"=w262:string)  [unwired: 1 out]
        n88 = for {
          tunnel: w262 -> [w274]
          tunnel: w261 -> [w272] mode=indexing
          tunnel: [w272] -> w258 mode=indexing if=w271
          n89 = Index Array(array=w272) -> (element=w273:string)  [unwired: 1 in]
          n90 = Equal?(x=w274, y=w273) -> (x = y?=w271:bool)
        }
        n91 = Bundle By Name(cluster=w260, "Test Limits"=w258) -> (w259:T5)
        n92 = call <vilib>:"Add State(s) to Queue__jki_lib_state_machine.vi"("State(s) in (\"\")"=w270) -> ("States Out"=w269:string)  [unwired: 14 in]
      }
      frame "Limits Test: Read Wait for Start Test" {
        w280 = "Read Wait for Start Test"  # Sub Test Name
        # "UDP Read Test = if equal to F0 = pass else fail"
        # "#Limits Testing - Add the sub test name for\ntest included in limits file"
        n93 = Unbundle By Name(w279) -> ("Test Limits"=w281:string[][], "Read Wait for Start"=w285:string)
        n94 = Unbundle By Name(w279) -> ("Results Data Array"=w277:string[][])
        n95 = To Variant(anything=w285) -> (Variant=w282:variant)
        n96 = call "Process Results.vi"("error in (no error)"=w283, "Measurement"=w282, "Test Limits"=w281, "Sub Test Name"=w280) -> ("error out"=w284:errorcluster, "Results Data"=w275:string[])  [unwired: 6 in]
        "Results Data 9" <- w275
        n97 = Build Array (concatenate)(w277, w275) -> (w276:string[][])
        n98 = Bundle By Name(cluster=w279, "Results Data Array"=w276) -> (w278:T5)
        n99 = call <vilib>:"Add State(s) to Queue__jki_lib_state_machine.vi"("State(s) in (\"\")"=w287) -> ("States Out"=w286:string)  [unwired: 14 in]
      }
      frame "Limits Test: Read Normal Operation Test" {
        w293 = "Read Normal Operation Test"  # Sub Test Name
        # "UDP Read Test = if equal to F0 = pass else fail"
        # "#Limits Testing - Add the sub test name for\ntest included in limits file"
        n100 = Unbundle By Name(w292) -> ("Test Limits"=w294:string[][], "Read Normal Operation"=w298:string)
        n101 = Unbundle By Name(w292) -> ("Results Data Array"=w290:string[][])
        n102 = To Variant(anything=w298) -> (Variant=w295:variant)
        n103 = call "Process Results.vi"("error in (no error)"=w296, "Measurement"=w295, "Test Limits"=w294, "Sub Test Name"=w293) -> ("error out"=w297:errorcluster, "Results Data"=w288:string[])  [unwired: 6 in]
        "Results Data 10" <- w288
        n104 = Build Array (concatenate)(w290, w288) -> (w289:string[][])
        n105 = Bundle By Name(cluster=w292, "Results Data Array"=w289) -> (w291:T5)
        n106 = call <vilib>:"Add State(s) to Queue__jki_lib_state_machine.vi"("State(s) in (\"\")"=w300) -> ("States Out"=w299:string)  [unwired: 14 in]
      }
      frame "---------- Results Data ----------" {
        # "Template Separator\n(You can make a copy of, or modify, this frame)"
        n107 = call <vilib>:"Add State(s) to Queue__jki_lib_state_machine.vi"("State(s) in (\"\")"=w304) -> ("States Out"=w303:string)  [unwired: 14 in]
      }
      frame "Results Data: Write Results Data" {
        w306 = ","  # delimiter (\t)
        w307 = TRUE  # append to file? (new file:F)
        n108 = Unbundle By Name(w309) -> ("Results File Path"=w308:path, "Results Data Array"=w305:string[][])
        "Results Data Array" <- w305
        n109 = call-poly <vilib>:"Write Delimited Spreadsheet.vi"("file path (dialog if empty)"=w308, "2D data"=w305, "append to file? (new file:F)"=w307, "error in (no error)"=w310, "delimiter (\\t)"=w306) -> ("error out"=w311:errorcluster)  [unwired: 9 in, 1 out]
        n110 = call <vilib>:"Add State(s) to Queue__jki_lib_state_machine.vi"("State(s) in (\"\")"=w313) -> ("States Out"=w312:string)  [unwired: 14 in]
      }
      frame "---------- Init ----------" {
        # "Template Separator\n(You can make a copy of, or modify, this frame)"
        n111 = call <vilib>:"Add State(s) to Queue__jki_lib_state_machine.vi"("State(s) in (\"\")"=w317) -> ("States Out"=w316:string)  [unwired: 14 in]
      }
      frame "Init: UDP Open" {
        # "Template Separator\n(You can make a copy of, or modify, this frame)"
        # "Open UDP linking to RIB Box."
        n112 = call "FGV - Initialise.vi"("Enum"=FGV_-_Enum."Get Data", "Error In"=w318) -> ("connection ID"=w319:refnum<k16>, "Error Out"=w320:errorcluster)  [unwired: 10 in, 2 out]
        n113 = Bundle By Name(cluster=w323, "connection ID"=w319) -> (w322:T5)
        n114 = call <vilib>:"Add State(s) to Queue__jki_lib_state_machine.vi"("State(s) in (\"\")"=w325) -> ("States Out"=w324:string)  [unwired: 14 in]
      }
      frame "Init: Start Timer (WfS)" {
        # "Start 10 second timer"
        # "Template Separator\n(You can make a copy of, or modify, this frame)"
        n115 = call "Timer.vi"("error in (no error)"=w332, "Target Time"=10.0, "Enum"=T4."Start Timer") -> ("error out"=w330:errorcluster)  [unwired: 5 in, 3 out]
        n116 = property on="Timeout (Wait for Start)" class="Slide (strict)"(error in=w330, "Value"=0.0 ("Horizontal Pointer Slide"), "Maximum"=10.0 ("Target Time"), "Minimum"=0.0 ("Scale.Range:Minimum")) -> (error out=w329:errorcluster)  [unwired: 1 in, 1 out]
        n117 = call <vilib>:"Add State(s) to Queue__jki_lib_state_machine.vi"("State(s) in (\"\")"=w336) -> ("States Out"=w335:string)  [unwired: 14 in]
      }
      frame "Init: Read Wait for Start State" {
        # "Read UDP if equal to F0 test complete if not check if timer has elapsed."
        # "#56 = didnt read before the timeout"
        # "Template Separator\n(You can make a copy of, or modify, this frame)"
        n118 = Unbundle By Name(w343) -> ("connection ID"=w356:refnum<k16>)
        n119 = UDP Read(connection ID=w356, timeout ms (25000)=1, 8:w338) -> (data out=w350:string, error out=w349:errorcluster, 3:w340:refnum<k16>)  [unwired: 1 in, 2 out]
        n120 = String Subset(string=w350, offset (0)=17 ("offset (0) 2"), length (rest)=1 ("length (rest) 2")) -> (substring=w352:string)
        n121 = String To Byte Array(string=w352) -> (unsigned byte array=w355:u8[])
        n122 = Number To Hexadecimal String(2:w355) -> (0:w354:string[])  [unwired: 1 in]
        n123 = Index Array(array=w354, index=0) -> (element=w344:string)
        n124 = Equal?(x=w344, y="15") -> (x = y?=w337:bool)
        "Wait for Start" <- w337
        n125 = call <vilib>:"Clear Errors.vi"("error in (no error)"=w349, "specific error code to clear (0: all)"=56) -> ("error out"=w339:errorcluster)  [unwired: 4 in, 1 out]
        n126 = Bundle By Name(cluster=w343, "connection ID"=w340, "Read Wait for Start"=w344) -> (w342:T5)
        n127 = call-poly <vilib>:"Select State(s)__jki_lib_state_machine.vi"("State(s) if True (\"\")"="Macro: Test 2" ("State(s) if True (\"\")"), "Select"=w337, "State(s) if False (\"\")"="Init: Elapsed Timer (WfS)" ("State(s) if False (\"\")")) -> ("States Out"=w341:string)  [unwired: 12 in]
        n128 = call <vilib>:"Add State(s) to Queue__jki_lib_state_machine.vi"("State(s) in Front (\"\")"=w341, "State(s) in (\"\")"=w360) -> ("States Out"=w359:string)  [unwired: 13 in]
      }
      frame "Init: Elapsed Timer (WfS)" {
        # "check if timer elased - if TRUE end test if FALSE read again."
        # "Template Separator\n(You can make a copy of, or modify, this frame)"
        # "Check to see if the timer has elpased."
        n129 = call "Timer.vi"("error in (no error)"=w368, "Target Time"=10.0, "Enum"=T4."Get Time") -> ("error out"=w367:errorcluster, "Time Elapsed?"=w364:bool, "Elapsed Time"=→"Timeout (Wait for Start)":dbl)  [unwired: 5 in, 1 out]
        n130 = call-poly <vilib>:"Select State(s)__jki_lib_state_machine.vi"("State(s) if True (\"\")"="Macro: Test 2" ("State(s) if True (\"\")"), "Select"=w364, "State(s) if False (\"\")"="Init: Read Wait for Start State" ("State(s) if False (\"\")")) -> ("States Out"=w363:string)  [unwired: 12 in]
        n131 = call <vilib>:"Add State(s) to Queue__jki_lib_state_machine.vi"("State(s) in Front (\"\")"=w363, "State(s) in (\"\")"=w372) -> ("States Out"=w371:string)  [unwired: 13 in]
      }
      frame "Init: Start Command" {
        # "None"
        # "RIB Box IP"
        # "Data"
        # "Length"
        # "ID"
        # "Target"
        # "Type"
        # "Pkt ID"
        # "SET"
        # "Template Separator\n(You can make a copy of, or modify, this frame)"
        n132 = Unbundle By Name(w390) -> ("connection ID"=w378:refnum<k16>)
        n133 = Build Array(u8 91 ("element"), u8 1 ("element"), u8 9 ("element"), u8 110 ("element"), u8 0 ("element")) -> (w388:u8[])
        n134 = Byte Array To String(unsigned byte array=w388) -> (string=w389:string)
        n135 = String To IP(1:"192.168.201.21" ("name")) -> (0:w381:u32)
        n136 = UDP Write(address=w381, port or service name=u16 54321, connection ID=w378, data in=w389, 8:w379, 9:1000 ("timeout ms (25000)")) -> (error out=w375:errorcluster, 3:w377:refnum<k16>)
        n137 = Bundle By Name(cluster=w390, "connection ID"=w377) -> (w391:T5)
        n138 = call <userlib>:"Wait (ms)__ogtk.vi"("error in (no error)"=w375, "milliseconds to wait"=u32 10000) -> ("error out"=w374:errorcluster)  [unwired: 8 in, 1 out]
        n139 = call <vilib>:"Add State(s) to Queue__jki_lib_state_machine.vi"("State(s) in (\"\")"=w393) -> ("States Out"=w392:string)  [unwired: 14 in]
      }
      frame "Init: Start Timer (Normal Op)" {
        # "Start 10 second timer"
        # "Template Separator\n(You can make a copy of, or modify, this frame)"
        n140 = call "Timer.vi"("error in (no error)"=w400, "Target Time"=10.0, "Enum"=T4."Start Timer") -> ("error out"=w397:errorcluster)  [unwired: 5 in, 3 out]
        n141 = property on="Timeout (Normal Operation)" class="Slide (strict)"(error in=w397, "Value"=0.0 ("Horizontal Pointer Slide"), "Maximum"=10.0 ("Target Time"), "Minimum"=0.0 ("Scale.Range:Minimum")) -> (error out=w398:errorcluster)  [unwired: 1 in, 1 out]
        n142 = call <vilib>:"Add State(s) to Queue__jki_lib_state_machine.vi"("State(s) in (\"\")"=w404) -> ("States Out"=w403:string)  [unwired: 14 in]
      }
      frame "Init: Read Normal Operation" {
        # "Read UDP if equal to F0 test complete if not check if timer has elapsed."
        # "#56 = didnt read before the timeout"
        # "Template Separator\n(You can make a copy of, or modify, this frame)"
        n143 = Unbundle By Name(w423) -> ("connection ID"=w426:refnum<k16>)
        n144 = UDP Read(connection ID=w426, timeout ms (25000)=1, 8:w422) -> (data out=w416:string, error out=w425:errorcluster, 3:w418:refnum<k16>)  [unwired: 1 in, 2 out]
        n145 = String Subset(string=w416, offset (0)=17 ("offset (0) 2"), length (rest)=1 ("length (rest) 2")) -> (substring=w415:string)
        n146 = String To Byte Array(string=w415) -> (unsigned byte array=w413:u8[])
        n147 = Number To Hexadecimal String(2:w413) -> (0:w414:string[])  [unwired: 1 in]
        n148 = Index Array(array=w414, index=0) -> (element=w419:string)
        n149 = Equal?(x=w419, y="19") -> (x = y?=w406:bool)
        "Normal Operation" <- w406
        n150 = Bundle By Name(cluster=w423, "connection ID"=w418, "Read Normal Operation"=w419) -> (w420:T5)
        n151 = call-poly <vilib>:"Select State(s)__jki_lib_state_machine.vi"("State(s) if True (\"\")"="Macro: Limits" ("State(s) if True (\"\")"), "Select"=w406, "State(s) if False (\"\")"="Init: Elapsed Timer (Normal Op)" ("State(s) if False (\"\")")) -> ("States Out"=w405:string)  [unwired: 12 in]
        n152 = call <vilib>:"Clear Errors.vi"("error in (no error)"=w425, "specific error code to clear (0: all)"=56) -> ("error out"=w421:errorcluster)  [unwired: 4 in, 1 out]
        n153 = call <vilib>:"Add State(s) to Queue__jki_lib_state_machine.vi"("State(s) in Front (\"\")"=w405, "State(s) in (\"\")"=w428) -> ("States Out"=w427:string)  [unwired: 13 in]
      }
      frame "Init: Elapsed Timer (Normal Op)" {
        # "check if timer elased - if TRUE end test if FALSE read again."
        # "Template Separator\n(You can make a copy of, or modify, this frame)"
        # "Check to see if the timer has elpased."
        n154 = call "Timer.vi"("error in (no error)"=w436, "Target Time"=10.0, "Enum"=T4."Get Time") -> ("error out"=w435:errorcluster, "Time Elapsed?"=w432:bool, "Elapsed Time"=→"Timeout (Normal Operation)":dbl)  [unwired: 5 in, 1 out]
        n155 = call-poly <vilib>:"Select State(s)__jki_lib_state_machine.vi"("State(s) if True (\"\")"="Macro: Limits" ("State(s) if True (\"\")"), "Select"=w432, "State(s) if False (\"\")"="Init: Read Normal Operation" ("State(s) if False (\"\")")) -> ("States Out"=w431:string)  [unwired: 12 in]
        n156 = call <vilib>:"Add State(s) to Queue__jki_lib_state_machine.vi"("State(s) in Front (\"\")"=w431, "State(s) in (\"\")"=w440) -> ("States Out"=w439:string)  [unwired: 13 in]
      }
    }
    n157 = Wait (ms)(milliseconds to wait=u32 2) -> ()  [unwired: 1 out]
  }
  "error out" <- w1
